vi "Randomize Color.vi"(0 "Color In":u32(colorbox)=16711680, 11 "error in (no error)":errorcluster) -> (4 "Randomized Color":u32(colorbox), 15 "error out":errorcluster)   [LabVIEW 2012]
doc: "This VI generates a random color. If you wire a color to \"Color In\" it will generate a random color of the same lightness and saturation, to maintain visual consistancy when used with another color.\n\nSee HSLToolsAdvancedExample.vi in the NI Example Finder for more information."
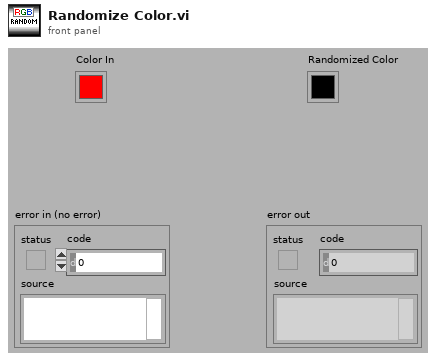
[diagram p1: front panel]
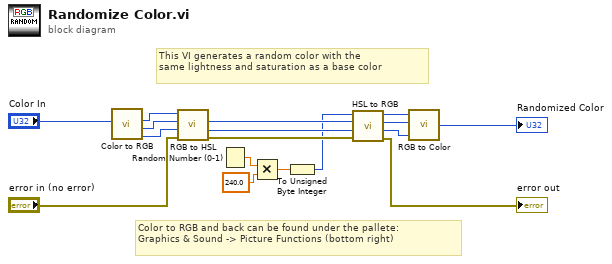
[diagram p0: block diagram]
diagram:
  # "This VI generates a random color with the\nsame lightness and saturation as a base color"
  # "Color to RGB and back can be found under the pallete:\nGraphics & Sound -> Picture Functions (bottom right)"
  n1 = call <vilib>:"Color to RGB.vi"("Color"="Color In") -> ("R"=w17:u8, "G"=w16:u8, "B"=w15:u8)  [unwired: 1 out]
  n2 = call <vilib>:"RGB to HSL.vi"("Error In"="error in (no error)", "Blue"=w15, "Green"=w16, "Red"=w17) -> ("Error Out"=w11:errorcluster, "Lum"=w5:u8, "Sat"=w10:u8)  [unwired: 5 out]
  n3 = Random Number (0-1)() -> (number: 0 to 1=w3:dbl)
  n4 = Multiply(x=w3, y=240.0) -> (x*y=w1:dbl)
  n5 = To Unsigned Byte Integer(number=w1) -> (unsigned 8bit integer=w4:u8)
  n6 = call <vilib>:"HSL to RGB.vi"("Error In"=w11, "Lum"=w5, "Sat"=w10, "Hue"=w4) -> ("Error Out"=→"error out":errorcluster, "Blue"=w12:u8, "Green"=w13:u8, "Red"=w14:u8)  [unwired: 4 out]
  n7 = call <vilib>:"RGB to Color.vi"("B"=w12, "G"=w13, "R"=w14) -> ("Color"=→"Randomized Color":u32)
